vi "FollowALine.vi"() -> ()   [LabVIEW 2016, in "LEGO-PMR.lvrbt"]
uses:
  LEGO-PMR.lvrbt
  <vilib>/NXT/Block Support/NXT_OutputPort.ctl
  <vilib>/NXT/Block Support/NXT_InputPort.ctl
  <vilib>/NXT/Dual Mode Library/Sensors/EV3_Color_Reflect.vi
  <vilib>/NXT/Dual Mode Library/Waits/Wait_Num(msec).vi
  <vilib>/NXT/NXTIO Xnodes/NXTIONodeSubVIs/NXTMoveMotors.vi
  <vilib>/NXT/NXTIO Xnodes/NXTIONodeSubVIs/NXTStopMotors.vi
  <vilib>/NXT/NXTIO Xnodes/AddressXNode/NXTIOAddress.xnode
  <vilib>/NXT/NXTIO Xnodes/NXTIOXNode/NXTIO.xnode
  <vilib>/NXT/Subs/LVHSConnector.ctl
  <vilib>/NXT/LegoClasses/BrickReference/BrickReference.lvclass
panel:
  out "Waveform Chart":sgl(graph)
  out "Light sensor readings":dbl
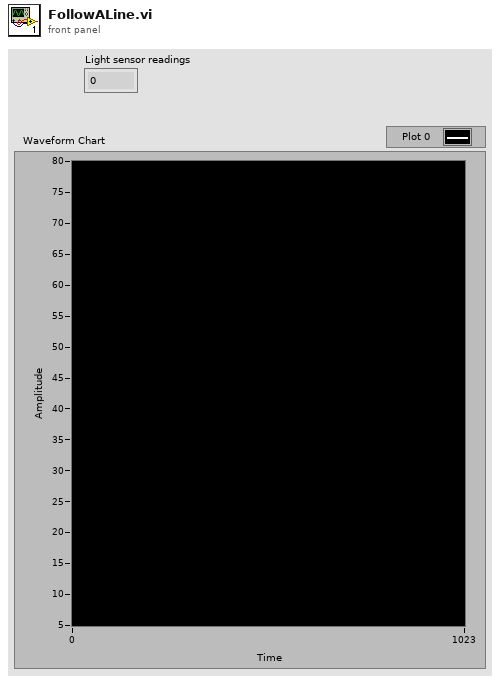
[diagram p1: front panel]
types:
  T1 = typedef "NXT_OutputPort.ctl" = u8
  T2 = typedef "NXT_InputPort.ctl" = u32
  T3 = typedef "LVHSConnector.ctl" = refnum<class "BrickReference.lvclass">
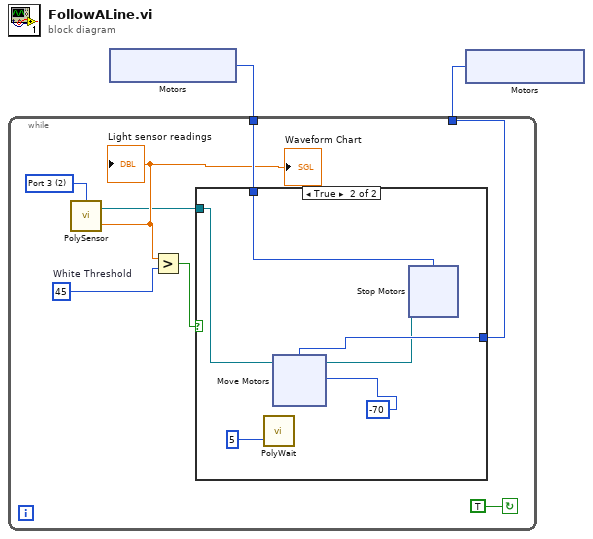
[diagram p0: block diagram]
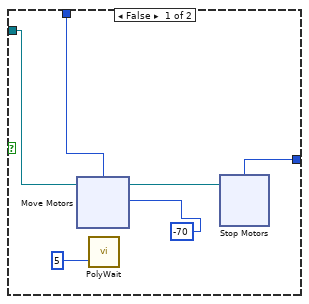
[diagram p2: hidden frame]
diagram:
  n1 = xnode "Motors"() -> ("Motor"=w1:T1)
  n2 = xnode "Motors"() -> ("Motor"=w2:T1)
  n3 = while {
    tunnel: w2 -> [w4]
    tunnel: w1 -> [w6]
    stop <- TRUE continue-if-true
    w8 = 45  # White Threshold
    w10 = T2 2 items=["Port 1", "Port 2", "Port 3", "Port 4"] ("Input Port (Port 3)")
    n4 = call-poly <vilib>:"PolySensor.vi"("Port (Port 1)"=w10) -> ("Scaled Value"=w5:sgl, "NXT/EV3"=w3:T3)  [unwired: 1 in, 1 out]
    "Light sensor readings" <- w5
    "Waveform Chart" <- w5
    n5 = Greater?(x=w5, y=w8) -> (0:w7:bool)
    n6 = case shown="True" w7 {
      tunnel: w6 -> [w15 w33]
      tunnel: w4 -> [w14 w32]
      tunnel: w3 -> [w13 w31]
      frame False {
        n7 = xnode "Move Motors"("Power/Speed 1"=-70, "Motors"=w15, "NXT/EV3"=w13) -> ("NXT/EV3"=w12:T3)
        n8 = call-poly <vilib>:"PolyWait.vi"("Time (100 msec)"=u32 5 ("Time (1 sec)")) -> ()  [unwired: 3 in, 1 out]
        n9 = xnode "Stop Motors"("Motors"=w14, "NXT/EV3"=w12) -> ()  [unwired: 1 out]
      }
      frame True {
        n10 = call-poly <vilib>:"PolyWait.vi"("Time (100 msec)"=u32 5 ("Time (1 sec)")) -> ()  [unwired: 3 in, 1 out]
        n11 = xnode "Move Motors"("Power/Speed 1"=-70, "Motors"=w32, "NXT/EV3"=w31) -> ("NXT/EV3"=w30:T3)
        n12 = xnode "Stop Motors"("Motors"=w33, "NXT/EV3"=w30) -> ()  [unwired: 1 out]
      }
    }
  }
